vi "myRIO_BRig_RT_dataExp_Tcycle_Reward_max_L.vi"() -> (2 "output_Tcycle_Reward_max_L":i32)   [LabVIEW 2014]
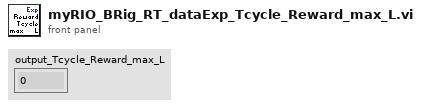
[diagram p1: front panel]
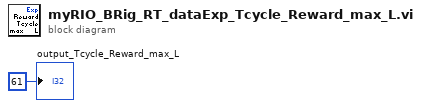
[diagram p0: block diagram]
diagram:
  "output_Tcycle_Reward_max_L" <- 61 ("output_iBlock")
